vi "Fit Spline to Velocity Profile2.vi"(9 "vel positions":sgl[](array[numeric]), 10 "s(t)":dbl[](array[numeric]), 11 "bezier spline":T1) -> ()   [LabVIEW 2019]
uses:
  Types/Bezier Spline.ctl
panel:
  in  "t":sgl[](array[numeric])
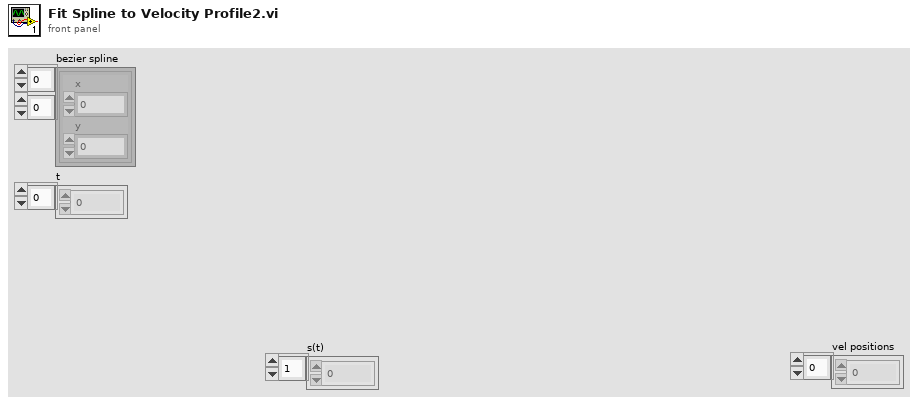
[diagram p1: front panel]
types:
  T1 = typedef "Bezier Spline.ctl" = cluster{"x":sgl, "y":sgl}[][]
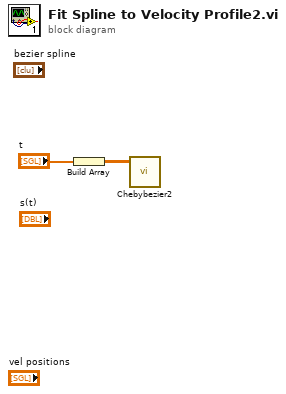
[diagram p0: block diagram]
diagram:
  n1 = Build Array("t") -> (w2:sgl[][])
  n2 = call "Chebybezier2.vi"("Y"=w2) -> ()  [unwired: 10 in, 1 out]
